vi "Active Pressure Compensation System.vi"() -> ()   [LabVIEW 2020]
uses:
  <vilib>/Instr/_visa.llb/VISA Configure Serial Port (Instr).vi
  <vilib>/addons/Fuzzy Logic/FL Fuzzy Controller (SISO).vi
  <vilib>/addons/Fuzzy Logic/NI_Fuzzy_Logic_API.lvlib
panel:
  out "Fuzzy Input":dbl
  in  "Setpoint Pressure Difference":dbl
  out "Defuzzification value":dbl
  out "Valve Direction":string="R"
  out "Pressurized      Released":bool=TRUE
  in  "byte count":u32(slide)=15 scale=0.0..50.0
  out "Pressure Difference":dbl=82.0
  in  "stop":bool
  out "STM32 Serial Read":string="82.00\r\n"
  in  "VISA resource name":refnum<visa-resource-name>="COM3"
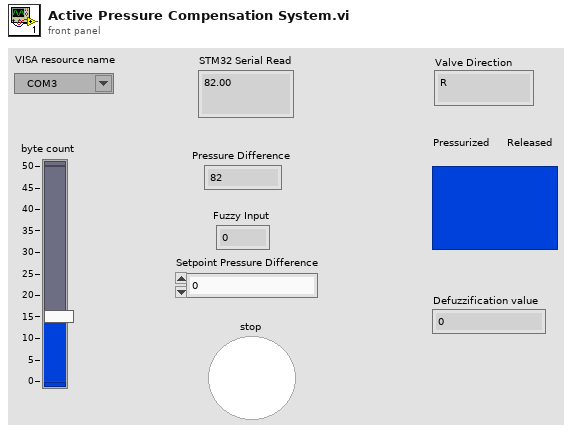
[diagram p1: front panel]
types:
  T1 = typedef "NI_Fuzzy_Logic_API.lvlib/FL System.ctl" = cluster{"input variables":T2[], "output variables":T2[], "rules":T5[], "defuzzification method":T11, "description":string, "user MF interpolating polynomials":T12[]}
  T2 = typedef "NI_Fuzzy_Logic_API.lvlib/FL Variable.ctl" = cluster{"name":string, "range":dbl[], "MFs":T3[]}
  T3 = typedef "NI_Fuzzy_Logic_API.lvlib/FL Membership Function.ctl" = cluster{"name":string, "shape":T4, "points":dbl[], "color":u32, "user-defined shape index":i32}
  T4 = typedef "NI_Fuzzy_Logic_API.lvlib/FL Membership Function Shape.ctl" = u16
  T5 = typedef "NI_Fuzzy_Logic_API.lvlib/FL Rule.ctl" = cluster{"antecedents":T6[], "antecedent connective":T8, "consequents":T9[], "consequent implication":T10, "degree of support":dbl}
  T6 = typedef "NI_Fuzzy_Logic_API.lvlib/FL Antecedent.ctl" = cluster{"Var Index":i32, "MF Index":i32, "Cond":T7}
  T7 = typedef "NI_Fuzzy_Logic_API.lvlib/FL Modifier.ctl" = u16
  T8 = typedef "NI_Fuzzy_Logic_API.lvlib/FL Antecedent Connective.ctl" = u16
  T9 = typedef "NI_Fuzzy_Logic_API.lvlib/FL Consequent.ctl" = cluster{"Var Index":i32, "MF Index":i32, "Cond":T7}
  T10 = typedef "NI_Fuzzy_Logic_API.lvlib/FL Consequent Implication.ctl" = u16
  T11 = typedef "NI_Fuzzy_Logic_API.lvlib/FL Defuzzification.ctl" = u16
  T12 = typedef "NI_Fuzzy_Logic_API.lvlib/FL Interpolating polynomials.ctl" = cluster{"X":dbl[], "Y":dbl[], "Y(x) coeff":dbl[][], "X(y) coeff":dbl[][], "Area(y) coeff":dbl[][], "coa_x(y) coeff":dbl[][]}
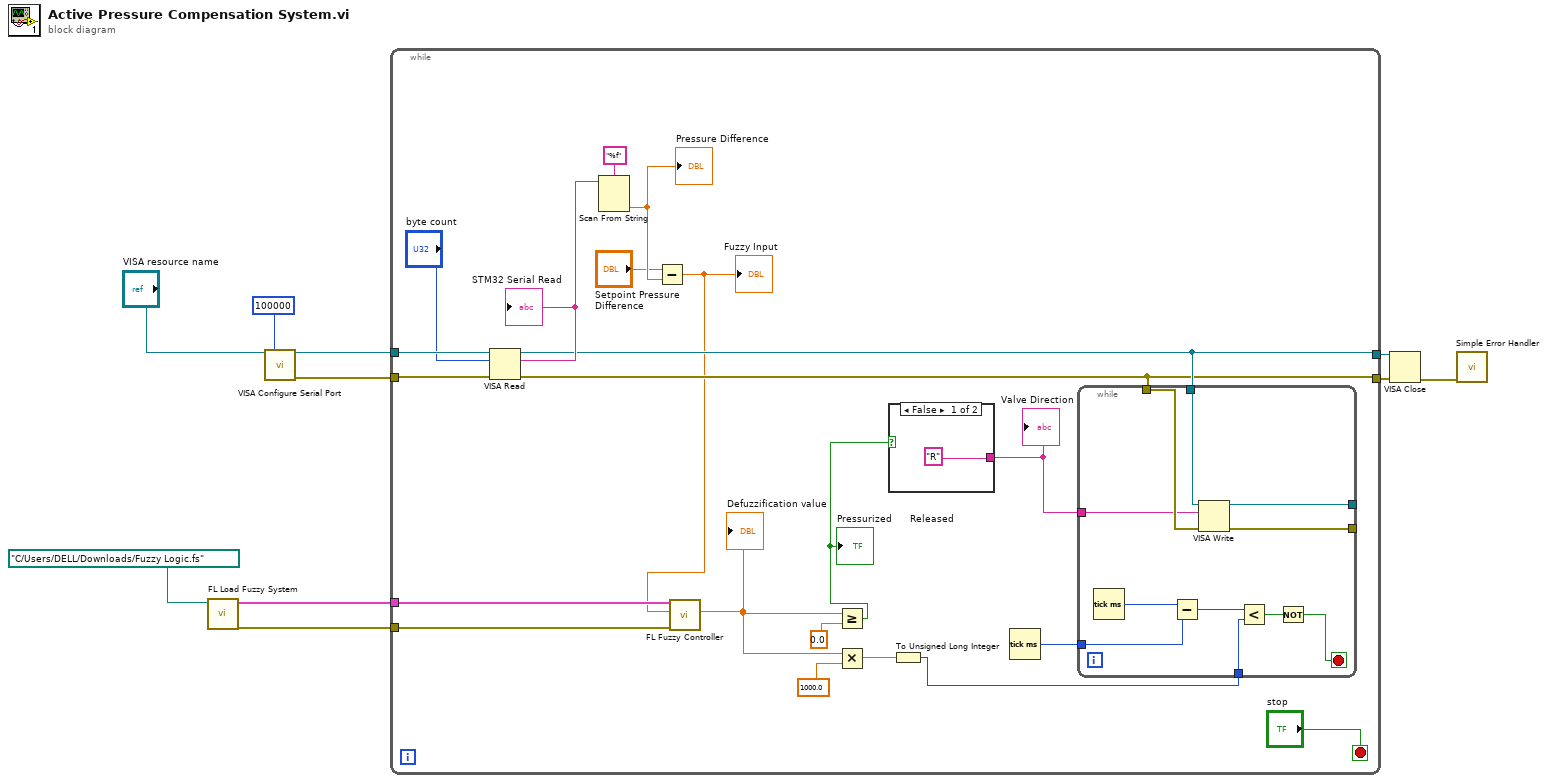
[diagram p0: block diagram]
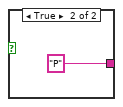
[diagram p2: hidden frame]
diagram:
  n1 = call <vilib>:"FL Load Fuzzy System.vi"("file path"=path "C:/Users/DELL/Downloads/Fuzzy Logic.fs") -> ("error out"=w2:errorcluster, "fuzzy system out"=w3:T1)  [unwired: 9 in]
  n2 = call-poly "VISA Configure Serial Port"("VISA resource name"="VISA resource name", "timeout (10sec)"=u32 100000) -> ("VISA resource name out"=w10:refnum<visa-resource-name>, "error out"=w8:errorcluster)  [unwired: 12 in]
  n3 = while {
    tunnel: w10 -> [w26]
    tunnel: [w21] -> w9
    tunnel: w8 -> [w25]
    tunnel: [w20] -> w7
    tunnel: w3 -> [w28]
    tunnel: w2 -> [w27]
    stop <- "stop" stop-if-true
    n4 = VISA Read(VISA resource name=w26, byte count="byte count", error in (no error)=w25) -> (VISA resource name out=w21:refnum<visa-resource-name>, read buffer=w30:string, error out=w20:errorcluster)  [unwired: 1 out]
    "STM32 Serial Read" <- w30
    n5 = Scan From String(format string="%f", input string=w30) -> (output 1=w13:dbl)  [unwired: 3 in, 3 out]
    "Pressure Difference" <- w13
    n6 = Subtract(x="Setpoint Pressure Difference", y=w13) -> (x-y=w11:dbl)
    "Fuzzy Input" <- w11
    n7 = call-poly <vilib>:"FL Fuzzy Controller.vi"("error in (no error)"=w27, "input value"=w11, "fuzzy system in"=w28) -> ("output value"=w14:dbl)  [unwired: 4 in, 4 out]
    "Defuzzification value" <- w14
    n8 = Greater Or Equal?(x=w14, y=0.0) -> (x >= y?=w15:bool)
    "Pressurized      Released" <- w15
    n9 = Multiply(x=w14, y=1000.0) -> (x*y=w18:dbl)
    n10 = case shown="False" w15 {
      tunnel: ["R" "P"] -> w19
      frame False {
      }
      frame True {
      }
    }
    "Valve Direction" <- w19
    n11 = To Unsigned Long Integer(number=w18) -> (unsigned 32bit integer=w17:u32)
    n12 = Tick Count (ms)() -> (millisecond timer value=w22:u32)
    n13 = while {
      tunnel: [w42] -> _
      tunnel: [w41] -> _
      tunnel: w22 -> [w39]
      tunnel: w21 -> [w35]
      tunnel: w20 -> [w34]
      tunnel: w19 -> [w33]
      tunnel: w17 -> [w32]
      stop <- w36 stop-if-true
      n14 = Tick Count (ms)() -> (millisecond timer value=w40:u32)
      n15 = Subtract(x=w40, y=w39) -> (x-y=w38:u32)
      n16 = VISA Write(VISA resource name=w35, write buffer=w33, error in (no error)=w34) -> (VISA resource name out=w42:refnum<visa-resource-name>, error out=w41:errorcluster)  [unwired: 1 out]
      n17 = Less?(x=w38, y=w32) -> (x < y?=w37:bool)
      n18 = Not(x=w37) -> (.not. x?=w36:bool)
    }
  }
  n19 = VISA Close(VISA resource name=w9, error in (no error)=w7) -> (error out=w4:errorcluster)
  n20 = call <vilib>:"Simple Error Handler.vi"("error in (no error)"=w4) -> ()  [unwired: 4 in, 5 out]
